vi "Comms Port Ref.vi"(8 "baud rate (9600)":u32=57600, 11 "Telemetry COM Port":refnum<visa-resource-name>) -> (0 "error out":errorcluster, 3 "Comms Port Ref":refnum<visa-resource-name>)   [LabVIEW 2014]
uses:
  <vilib>/Instr/_visa.llb/VISA Flush IO Buffer Mask.ctl
  <vilib>/Instr/_visa.llb/VISA Configure Serial Port (Instr).vi
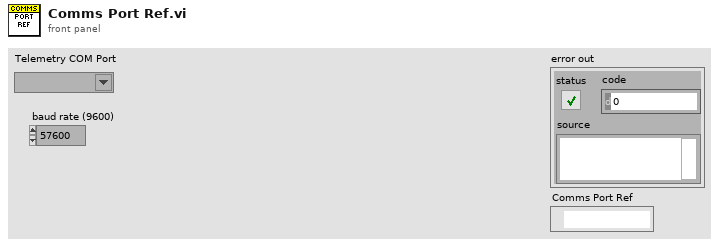
[diagram p1: front panel]
types:
  T1 = typedef "VISA Flush IO Buffer Mask.ctl" = u16
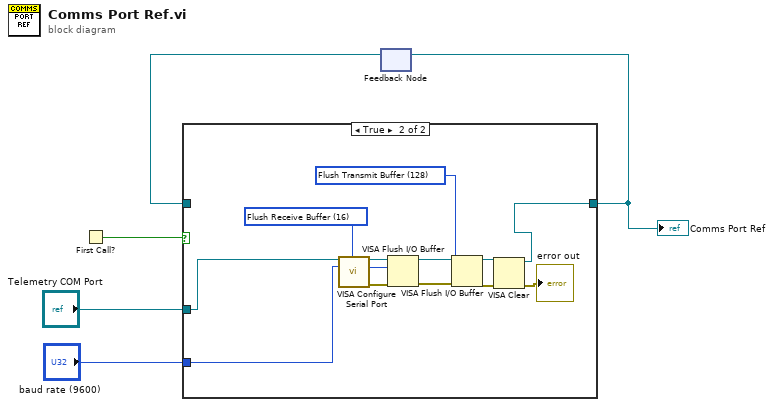
[diagram p0: block diagram]
diagram:
  n1 = First Call?() -> (First Call?: T/F=w1:bool)
  n2 = feedback #1() -> (w4:refnum<visa-resource-name>)  [unwired: 1 in]
  n3 = case shown="True" w1 {
    tunnel: [w6 w8] -> w5
    tunnel: w4 -> [w6 _]
    tunnel: "Telemetry COM Port" -> [_ w18]
    tunnel: "baud rate (9600)" -> [_ w17]
    frame False {
    }
    frame True {
      w11 = T1 128 items=["Flush Receive Buffer"=16, "Write Transmit Buffer to Device"=32, "Flush Receive Buffer (No I/O)"=64, "Flush Transmit Buffer"=128] ("Mask")
      w14 = T1 16 items=["Flush Receive Buffer"=16, "Write Transmit Buffer to Device"=32, "Flush Receive Buffer (No I/O)"=64, "Flush Transmit Buffer"=128] ("Mask")
      n4 = call-poly "VISA Configure Serial Port"("VISA resource name"=w18, "baud rate (9600)"=w17) -> ("VISA resource name out"=w16:refnum<visa-resource-name>, "error out"=w15:errorcluster)  [unwired: 12 in]
      n5 = VISA Flush I/O Buffer(VISA resource name=w16, mask (16)=w14, error in (no error)=w15) -> (VISA resource name out=w13:refnum<visa-resource-name>, error out=w12:errorcluster)
      n6 = VISA Flush I/O Buffer(VISA resource name=w13, mask (16)=w11, error in (no error)=w12) -> (VISA resource name out=w10:refnum<visa-resource-name>, error out=w9:errorcluster)
      n7 = VISA Clear(VISA resource name=w10, error in (no error)=w9) -> (VISA resource name out=w8:refnum<visa-resource-name>, error out=→"error out":errorcluster)
    }
  }
  "Comms Port Ref" <- w5
  n8 = feedback-in #1(w5) -> ()
